vi "SM_VDUT SEL.vi"(2 "error in (no error)":errorcluster, 3 "Port2 IN":u8 format="%x", 4 "Power Voltage":enum16{"+3.3V", "+5V"}(ring)) -> (0 "error out":errorcluster, 1 "Port2 OUT":u8 format="%x")   [LabVIEW 2011]
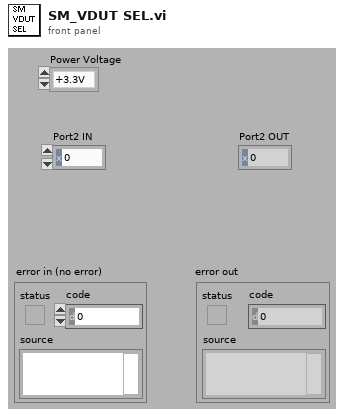
[diagram p1: front panel]
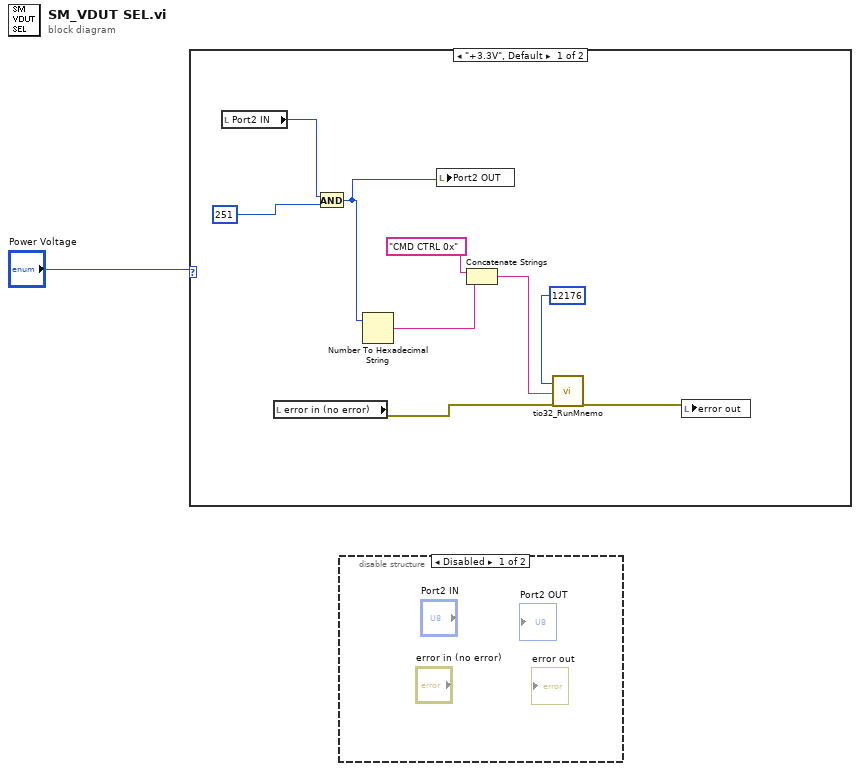
[diagram p0: block diagram]
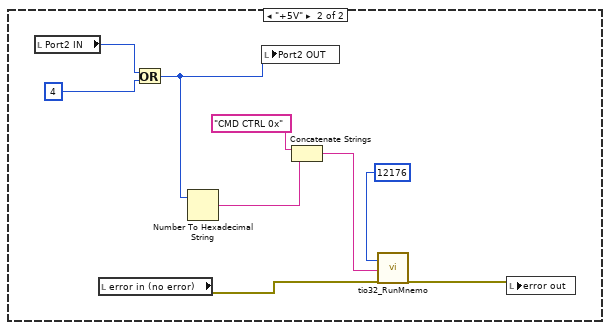
[diagram p3: hidden frame]
diagram:
  n1 = case shown="\"+3.3V\", Default" "Power Voltage" {
    frame "+3.3V", Default {
      n2 = local read "Port2 IN"() -> (w3:u8)
      n3 = local read "error in (no error)"() -> (w5:errorcluster)
      n4 = And(x=w3, y=u8 251) -> (x .and. y?=w2:u8)
      n5 = Number To Hexadecimal String(2:w2) -> (0:w6:string)  [unwired: 1 in]
      n6 = local write "Port2 OUT"(w2) -> ()
      n7 = Concatenate Strings("CMD CTRL 0x" ("command string"), w6) -> (w7:string)
      n8 = call "tio32_RunMnemo.vi"("Device address"=12176, "command string"=w7, "error in (no error)"=w5) -> ("error out"=w4:errorcluster)  [unwired: 6 in, 10 out]
      n9 = local write "error out"(w4) -> ()
    }
    frame "+5V" {
      n10 = local read "Port2 IN"() -> (w12:u8)
      n11 = local read "error in (no error)"() -> (w15:errorcluster)
      n12 = Or(x=w12, y=u8 4) -> (x .or. y?=w13:u8)
      n13 = Number To Hexadecimal String(2:w13) -> (0:w16:string)  [unwired: 1 in]
      n14 = local write "Port2 OUT"(w13) -> ()
      n15 = Concatenate Strings("CMD CTRL 0x" ("command string"), w16) -> (w17:string)
      n16 = call "tio32_RunMnemo.vi"("Device address"=12176, "command string"=w17, "error in (no error)"=w15) -> ("error out"=w14:errorcluster)  [unwired: 6 in, 10 out]
      n17 = local write "error out"(w14) -> ()
    }
  }
  n18 = disable-structure shown="Disabled" {
    frame Disabled {
    }
    frame Enabled {
    }
  }
